vi "GetState.vi"(8 "error in (no error)":errorcluster, 11 "Optics in":refnum<class "Optics.lvclass">) -> (0 "error out":errorcluster, 3 "Optics out":refnum<class "Optics.lvclass">)   [LabVIEW 2018, in "Optics.lvclass"]
uses:
  Optics.lvclass
  Optics.lvclass/Optics.ctl
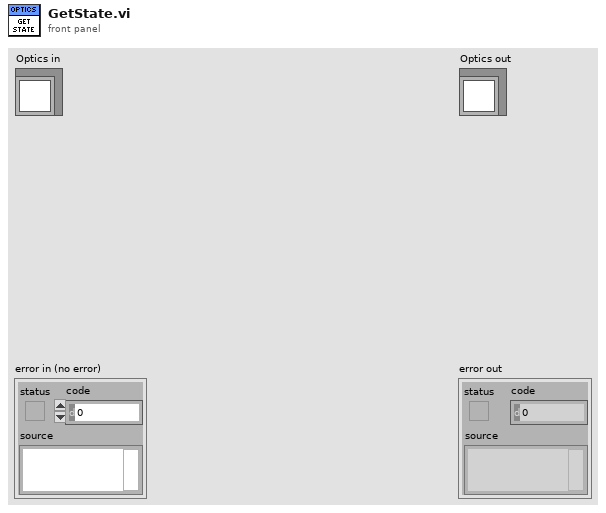
[diagram p1: front panel]
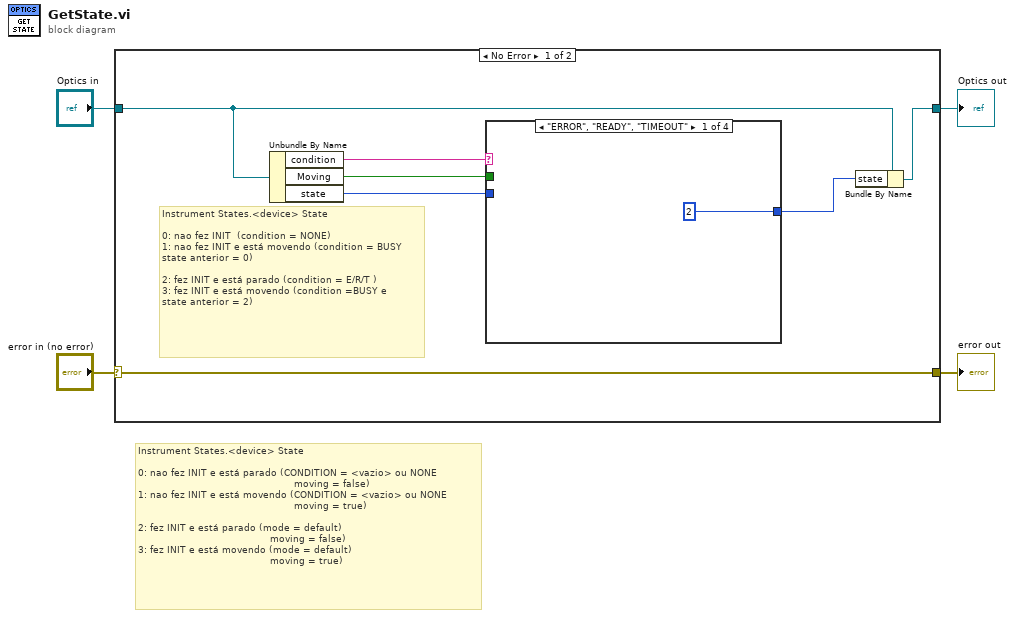
[diagram p0: block diagram]
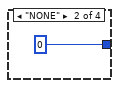
[diagram p2: hidden frame]
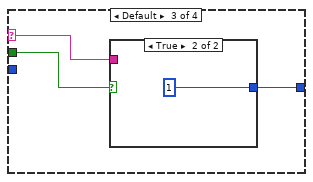
[diagram p3: hidden frame]
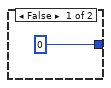
[diagram p4: hidden frame]
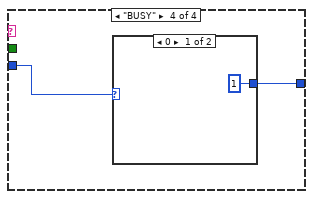
[diagram p5: hidden frame]
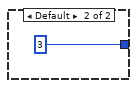
[diagram p6: hidden frame]
diagram:
  # "Instrument States.<device> State\n\n0: nao fez INIT e está parado (CONDITION = <vazio> ou NONE\n                                                    moving = false)\n1: nao fez INIT e está movendo (CONDITION = <vazio> ou NONE\n                                                    moving = true)\n\n2: fez INIT e está parado (mode = default)\n                                            moving = false)\n3: fez INIT e está movendo (mode = default)\n                                            moving = true)"
  n1 = case shown="No Error" "error in (no error)" {
    selector: "error in (no error)" -> [w11 w24]
    tunnel: [w11 w24] -> w3
    tunnel: [w6 w23] -> w1
    tunnel: "Optics in" -> [w8 w23]
    frame No Error {
      # "Instrument States.<device> State\n\n0: nao fez INIT  (condition = NONE)\n1: nao fez INIT e está movendo (condition = BUSY\nstate anterior = 0)\n\n2: fez INIT e está parado (condition = E/R/T )\n3: fez INIT e está movendo (condition =BUSY e \nstate anterior = 2)"
      n2 = Unbundle By Name(w8) -> ("condition"=w10:string, "Moving"=w9:bool, "state"=w5:u8)
      n3 = case shown="\"ERROR\", \"READY\", \"TIMEOUT\"" w10 {
        selector: w10 -> [_ _ w14 _]
        tunnel: [u8 2 u8 0 w16 w20] -> w7
        tunnel: w9 -> [_ _ w15 _]
        tunnel: w5 -> [_ _ _ w19]
        frame "ERROR", "READY", "TIMEOUT" {
        }
        frame "NONE" {
        }
        frame Default {
          n4 = case shown="True" w15 {
            tunnel: [u8 0 u8 1] -> w16
            tunnel: w14 -> [_ _]
            frame False {
            }
            frame True {
            }
          }
        }
        frame "BUSY" {
          n5 = case shown="0" w19 {
            tunnel: [u8 1 u8 3] -> w20
            frame 0 {
            }
            frame Default {
            }
          }
        }
      }
      n6 = Bundle By Name(cluster=w8, "state"=w7) -> (w6:refnum<class "Optics.lvclass">)
    }
    frame Error {
    }
  }
  "error out" <- w3
  "Optics out" <- w1
